vi "Tools Bar.vi"() -> ()   [LabVIEW 2017]
uses:
  widgets/EnumStateMachine.llb/Toolbar_Enum.ctl
  widgets/EnumStateMachine.llb/Main_Enum.ctl
  widgets/EnumStateMachine.llb/Toolbar_InsertQueue.vi
  widgets/EnumStateMachine.llb/Toolbar_RemoveQueue.vi
  widgets/EnumStateMachine.llb/Main_InsertQueue.vi
panel:
  in  "File Path Control":path
  in  "Save":bool
  in  "TB_Task":bool
  in  "TB_Alarm":bool
  in  "TB_Config":bool
  in  "TB_Stop":bool
  in  "TB_Run":bool
  in  "TB_Right":bool
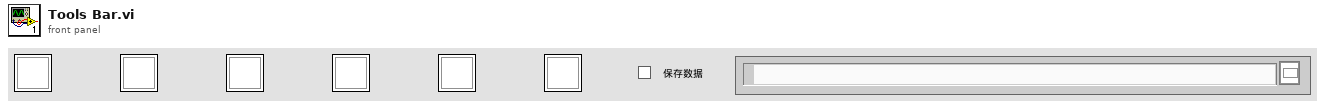
[diagram p1: front panel]
types:
  T1 = typedef "Toolbar_Enum.ctl" = enum16{"Core: Idle", "Core: Initialize", "Core: Error handle", "Core: Data prepare", "TB_Change", "Blinking_Alarm", "Chang_Save"}
  T2 = typedef "Queue RefNum" = refnum<k1>
  T3 = typedef "Main_Enum.ctl" = enum16{"Initialize", "SubPannel: Initialize", "Idel", "Show_Task infor", "Show_Daq config", "Run_Task", "Stop_Task", "Show_Alarm", "Show_Right", "Set_Save data", "Error handle", "Exit"}
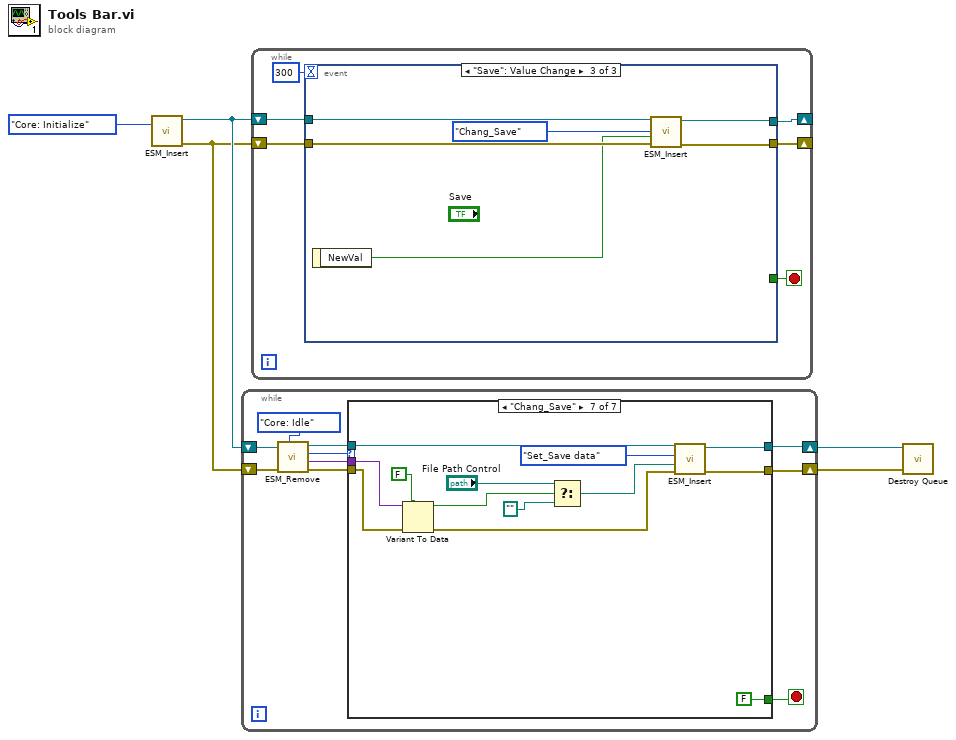
[diagram p0: block diagram]
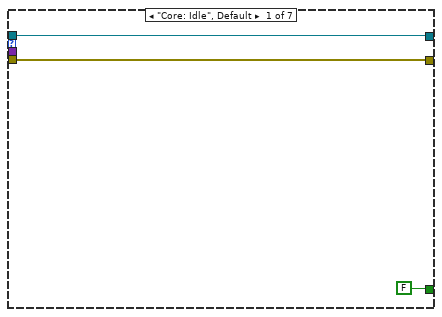
[diagram p2: hidden frame]
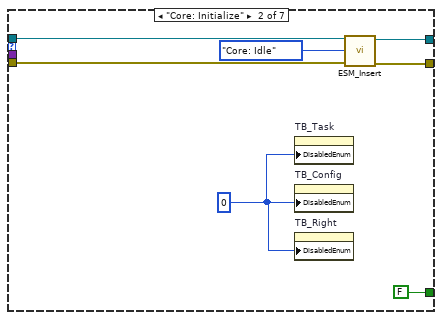
[diagram p3: hidden frame]
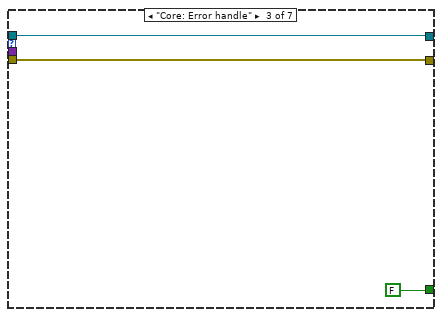
[diagram p4: hidden frame]
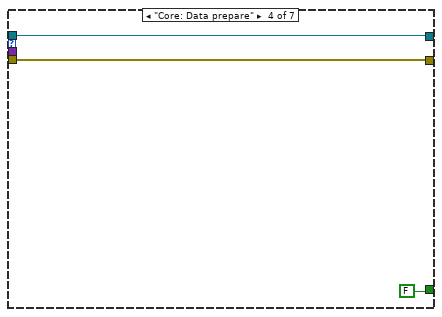
[diagram p5: hidden frame]
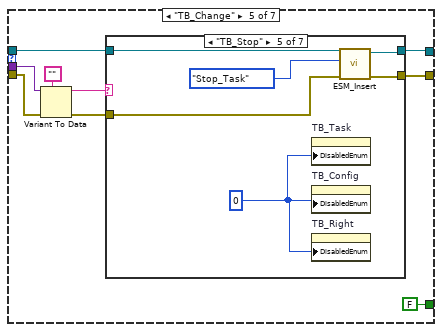
[diagram p6: hidden frame]
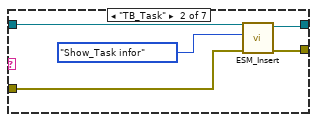
[diagram p8: hidden frame]
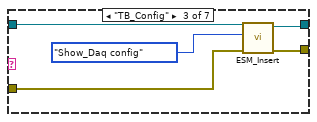
[diagram p9: hidden frame]
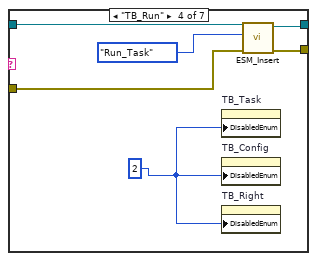
[diagram p10: hidden frame]
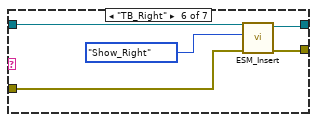
[diagram p11: hidden frame]
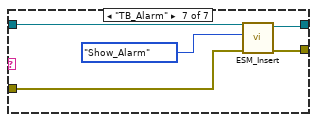
[diagram p12: hidden frame]
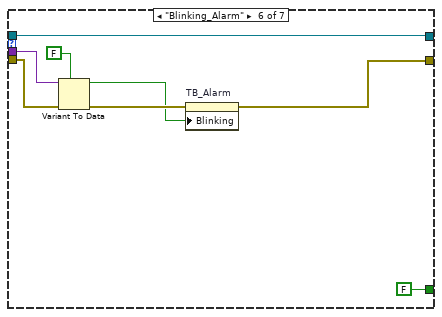
[diagram p13: hidden frame]
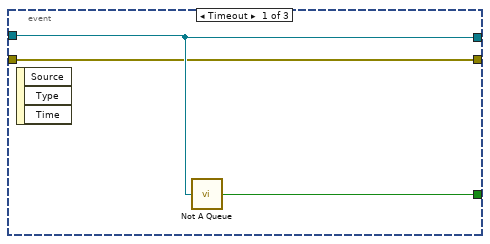
[diagram p14: hidden frame]
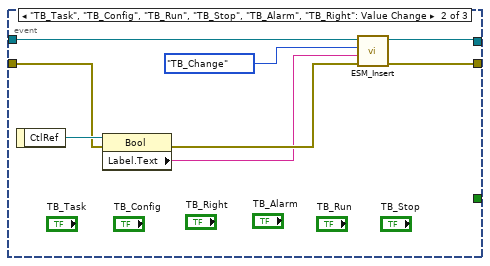
[diagram p15: hidden frame]
diagram:
  n1 = call-poly "ESM_Insert.vi"("Toolbar"=Toolbar_Enum."Core: Initialize") -> ("error out"=w3:errorcluster, "queue out"=w4:T2)  [unwired: 9 in]
  n2 = while {
    shift-right: [w8] -> w2
    shift-left: w4 -> [w15]
    shift-right: [w7] -> w1
    shift-left: w3 -> [w14]
    stop <- w6 stop-if-true
    n3 = call-poly "ESM_Remove.vi"("Default"=Toolbar_Enum."Core: Idle", "error in (no error)"=w14, "queue"=w15) -> ("错误输出"=w11:errorcluster, "data"=w10:variant, "Template out"=w12:T1, "queue out"=w9:T2)  [unwired: 5 in]
    n4 = case shown="\"Chang_Save\"" w12 {
      tunnel: w11 -> [w17 w24 w27 w30 w40 w80 w92]
      tunnel: w10 -> [_ _ _ _ w39 w79 w91]
      tunnel: w9 -> [w18 w25 w28 w31 w36 w82 w93]
      tunnel: [w18 w22 w28 w31 w35 w82 w95] -> w8
      tunnel: [w17 w21 w27 w30 w33 w76 w94] -> w7
      tunnel: [FALSE FALSE FALSE FALSE FALSE FALSE FALSE] -> w6
      frame "Core: Idle", Default {
      }
      frame "Core: Initialize" {
        w20 = 0
        n5 = property on="TB_Task" class="Bool"("DisabledEnum"=w20) -> ()  [unwired: 2 in, 2 out]
        n6 = property on="TB_Config" class="Bool"("DisabledEnum"=w20) -> ()  [unwired: 2 in, 2 out]
        n7 = property on="TB_Right" class="Bool"("DisabledEnum"=w20) -> ()  [unwired: 2 in, 2 out]
        n8 = call-poly "ESM_Insert.vi"("error in (no error)"=w24, "Toolbar"=Toolbar_Enum."Core: Idle", "queue"=w25) -> ("error out"=w21:errorcluster, "queue out"=w22:T2)  [unwired: 7 in]
      }
      frame "Core: Error handle" {
      }
      frame "Core: Data prepare" {
      }
      frame "TB_Change" {
        n9 = Variant To Data(error in=w40, type="", Variant=w39) -> (data=w37:string, error out=w34:errorcluster)
        n10 = case shown="\"TB_Stop\"" w37 {
          tunnel: w36 -> [w42 w46 w51 w57 w63 w68 w73]
          tunnel: [w42 w44 w49 w55 w61 w66 w71] -> w35
          tunnel: w34 -> [w41 w45 w50 w56 w62 w67 w72]
          tunnel: [w41 w47 w52 w58 w64 w69 w74] -> w33
          frame "", Default {
          }
          frame "TB_Task" {
            n11 = call-poly "ESM_Insert.vi"("error in (no error)"=w45, "Main"=Main_Enum."Show_Task infor", "queue"=w46) -> ("error out"=w47:errorcluster, "queue out"=w44:T2)  [unwired: 7 in]
          }
          frame "TB_Config" {
            n12 = call-poly "ESM_Insert.vi"("error in (no error)"=w50, "Main"=Main_Enum."Show_Daq config", "queue"=w51) -> ("error out"=w52:errorcluster, "queue out"=w49:T2)  [unwired: 7 in]
          }
          frame "TB_Run" {
            w53 = 2
            n13 = property on="TB_Task" class="Bool"("DisabledEnum"=w53) -> ()  [unwired: 2 in, 2 out]
            n14 = property on="TB_Config" class="Bool"("DisabledEnum"=w53) -> ()  [unwired: 2 in, 2 out]
            n15 = property on="TB_Right" class="Bool"("DisabledEnum"=w53) -> ()  [unwired: 2 in, 2 out]
            n16 = call-poly "ESM_Insert.vi"("error in (no error)"=w56, "Main"=Main_Enum."Run_Task", "queue"=w57) -> ("error out"=w58:errorcluster, "queue out"=w55:T2)  [unwired: 7 in]
          }
          frame "TB_Stop" {
            w59 = 0
            n17 = property on="TB_Task" class="Bool"("DisabledEnum"=w59) -> ()  [unwired: 2 in, 2 out]
            n18 = property on="TB_Config" class="Bool"("DisabledEnum"=w59) -> ()  [unwired: 2 in, 2 out]
            n19 = property on="TB_Right" class="Bool"("DisabledEnum"=w59) -> ()  [unwired: 2 in, 2 out]
            n20 = call-poly "ESM_Insert.vi"("error in (no error)"=w62, "Main"=Main_Enum."Stop_Task", "queue"=w63) -> ("error out"=w64:errorcluster, "queue out"=w61:T2)  [unwired: 7 in]
          }
          frame "TB_Right" {
            n21 = call-poly "ESM_Insert.vi"("error in (no error)"=w67, "Main"=Main_Enum."Show_Right", "queue"=w68) -> ("error out"=w69:errorcluster, "queue out"=w66:T2)  [unwired: 7 in]
          }
          frame "TB_Alarm" {
            n22 = call-poly "ESM_Insert.vi"("error in (no error)"=w72, "Main"=Main_Enum."Show_Alarm", "queue"=w73) -> ("error out"=w74:errorcluster, "queue out"=w71:T2)  [unwired: 7 in]
          }
        }
      }
      frame "Blinking_Alarm" {
        n23 = Variant To Data(error in=w80, type=FALSE, Variant=w79) -> (data=w75:bool, error out=w77:errorcluster)
        n24 = property on="TB_Alarm" class="Bool"(error in=w77, "Blinking"=w75) -> (error out=w76:errorcluster)  [unwired: 1 in, 1 out]
      }
      frame "Chang_Save" {
        n25 = Variant To Data(error in=w92, type=FALSE, Variant=w91) -> (data=w89:bool, error out=w87:errorcluster)
        n26 = Select(t="File Path Control", s=w89, f=path "") -> (s? t:f=w86:path)
        n27 = call-poly "ESM_Insert.vi"("error in (no error)"=w87, "data"=w86, "Main"=Main_Enum."Set_Save data", "queue"=w93) -> ("error out"=w94:errorcluster, "queue out"=w95:T2)  [unwired: 6 in]
      }
    }
  }
  n28 = while {
    shift-right: [w97] -> _
    shift-left: w4 -> [w101]
    shift-right: [w96] -> _
    shift-left: w3 -> [w100]
    stop <- w98 stop-if-true
    n29 = event shown="[2] \"Save\": Value Change" {
      selector: _ -> [_ _ _]
      dyn-events: _ -> [_ _ _]
      timeout: 300 -> [_ _ _]
      tunnel: w101 -> [w103 w110 w118]
      tunnel: w100 -> [w102 w111 w117]
      tunnel: [w104 _ _] -> w98
      tunnel: [w103 w109 w116] -> w97
      tunnel: [w102 w108 w115] -> w96
      event Timeout {
        n30 = event-data() -> ()  [unwired: 1 in, 3 out]
        n31 = call <vilib>:"Not A Queue.vi"("queue"=w103) -> ("is a queue?"=w104:bool)
      }
      event "TB_Task", "TB_Config", "TB_Run", "TB_Stop", "TB_Alarm", "TB_Right": Value Change {
        n32 = event-data() -> ("CtlRef"=w112:refnum<vi>)  [unwired: 1 in]
        n33 = property class="Bool"(reference=w112, error in=w111) -> (error out=w107:errorcluster, "Label.Text"=w106:string)  [unwired: 1 out]
        n34 = call-poly "ESM_Insert.vi"("error in (no error)"=w107, "data"=w106, "Toolbar"=Toolbar_Enum."TB_Change", "queue"=w110) -> ("error out"=w108:errorcluster, "queue out"=w109:T2)  [unwired: 6 in]
      }
      event "Save": Value Change {
        n35 = event-data() -> ("NewVal"=w114:bool)  [unwired: 1 in]
        n36 = call-poly "ESM_Insert.vi"("error in (no error)"=w117, "data"=w114, "Toolbar"=Toolbar_Enum."Chang_Save", "queue"=w118) -> ("error out"=w115:errorcluster, "queue out"=w116:T2)  [unwired: 6 in]
      }
    }
  }
  n37 = call <vilib>:"Destroy Queue.vi"("error in (no error)"=w1, "queue"=w2) -> ()  [unwired: 3 in, 3 out]
